vi "Connector Pane.vi"(8 "error in (no error)":errorcluster, 10 "Wire Middle? (F)":bool, 11 "VI Refnum in":refnum<vi>) -> (0 "error out":errorcluster, 3 "VI Refnum out":refnum<vi>)   [LabVIEW 2019, in "Builtins.lvlib"]
doc: "Wires the selected front panel controls and indicators to the connector pane ordered top-to-bottom then left-to-right respectively. Error In and Error Out terminals are wired to the bottom-left and bottom-right. All control terminals are set to Required inputs.\n\nCreated by: Ryan Pacini"
uses:
  Builtins.lvlib
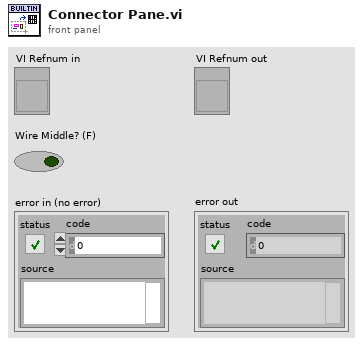
[diagram p1: front panel]
types:
  T1 = cluster{"Top":i16, "Left":i16, "Control":refnum<vi>}
  T2 = enum16{"Invalid Wire Rule", "Required", "Recommended", "Optional", "Dynamic Dispatch"}
  T3 = typedef "LVRectTypeDef.ctl" = cluster{"Left":i16, "Top":i16, "Right":i16, "Bottom":i16}
  T4 = cluster{"Top":i16, "Left":i16, "Control":refnum<vi>}[]
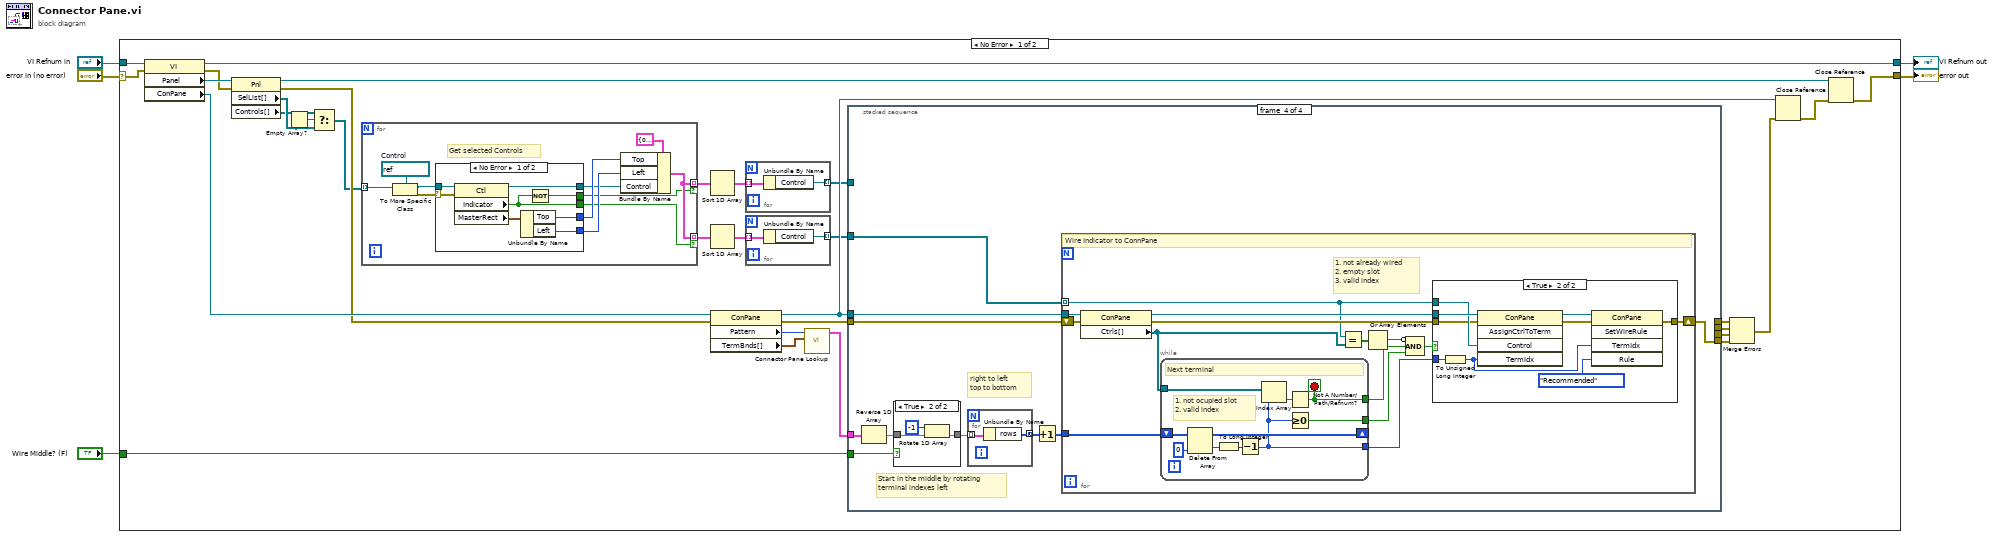
[diagram p0: block diagram]
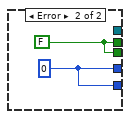
[diagram p2: hidden frame]
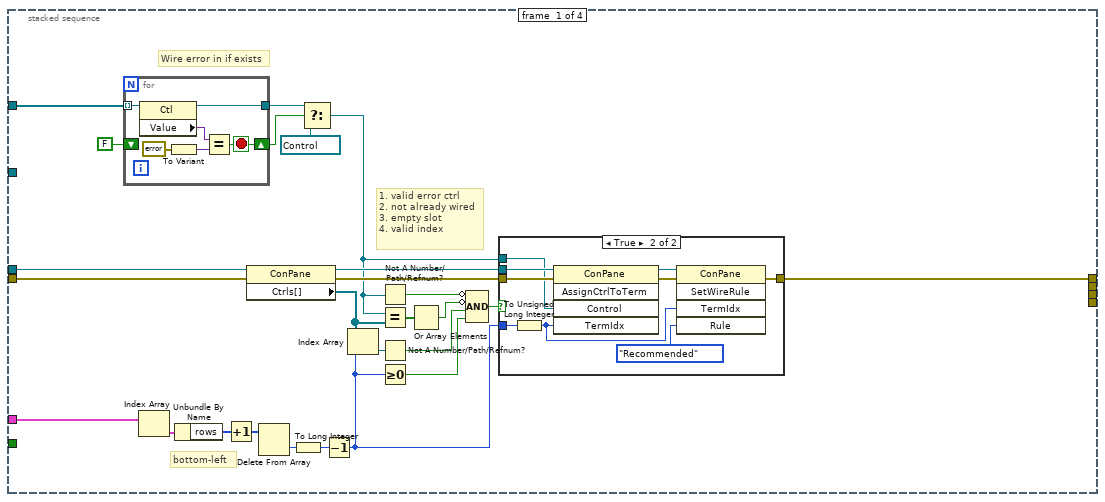
[diagram p3: hidden frame]
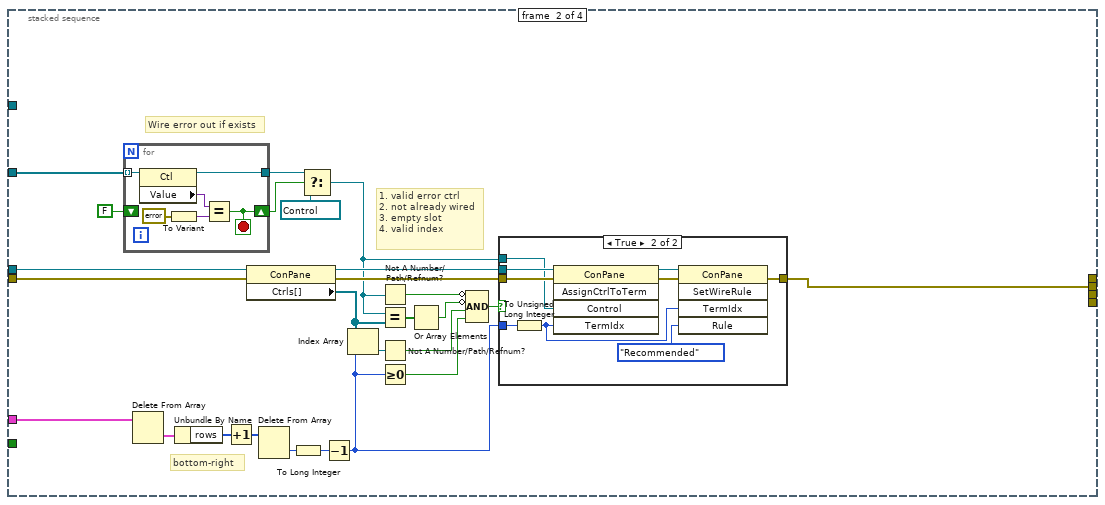
[diagram p5: hidden frame]
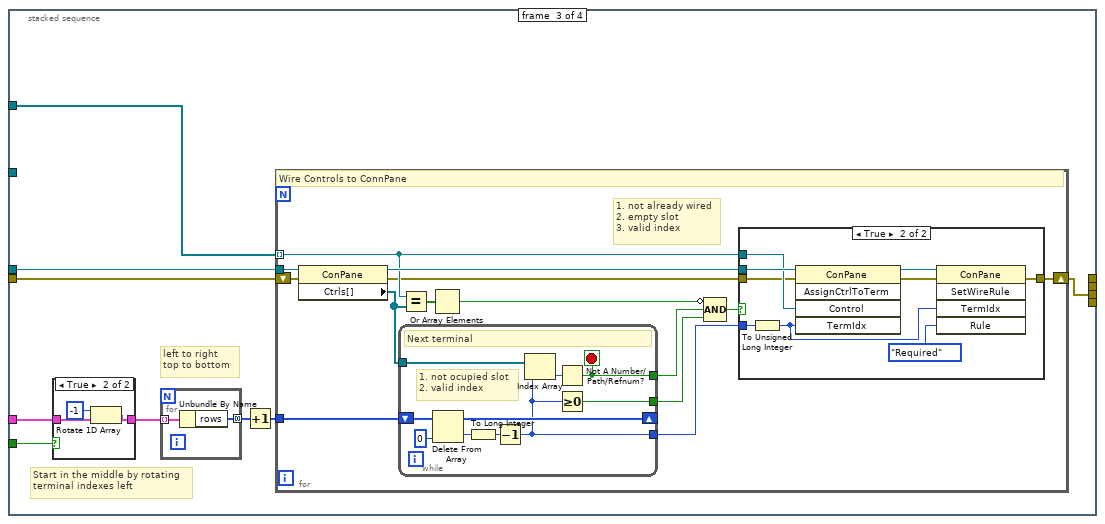
[diagram p7: hidden frame]
diagram:
  n1 = case shown="No Error" "error in (no error)" {
    selector: "error in (no error)" -> [w35 w245]
    tunnel: [w32 w246] -> w5
    tunnel: "VI Refnum in" -> [w36 w246]
    tunnel: [w18 w245] -> w2
    tunnel: "Wire Middle? (F)" -> [w6 _]
    frame No Error {
      n2 = property on="Property Node" class="VI"(reference=w36, error in=w35) -> (reference out=w32:refnum<vi>, error out=w33:errorcluster, "Panel"=w34:refnum<vi>, "ConPane"=w27:refnum<vi>)
      n3 = property on="Property Node" class="Pnl"(reference=w34, error in=w33) -> (reference out=w20:refnum<vi>, error out=w25:errorcluster, "SelList[]"=w10:refnum<vi>[], "Controls[]"=w9:refnum<vi>[])
      n4 = Empty Array?(array=w10) -> (empty?=w11:bool)
      n5 = Select(t=w9, s=w11, f=w10) -> (s? t:f=w8:refnum<vi>[])
      n6 = for {
        tunnel: w8 -> [w51] mode=indexing
        tunnel: [w46] -> w31 mode=indexing if=w43
        tunnel: [w46] -> w30 mode=indexing if=w42
        w50 = refnum<vi> refnum  # Control
        # "Get selected Controls"
        n7 = To More Specific Class(target class=w50, reference=w51) -> (specific class reference=w48:refnum<vi>, error out=w49:errorcluster)  [unwired: 1 in]
        n8 = case shown="No Error" w49 {
          selector: w49 -> [w52 _]
          tunnel: w48 -> [w59 _]
          tunnel: [w55 w61] -> w42
          tunnel: [w57 _] -> w41
          tunnel: [w56 w60] -> w47
          tunnel: [w54 w61] -> w43
          tunnel: [w53 w60] -> w44
          frame No Error {
            n9 = property class="Ctl"(reference=w59, error in=w52) -> (reference out=w57:refnum<vi>, "Indicator"=w55:bool, "MasterRect"=w58:T3)  [unwired: 1 out]
            n10 = Unbundle By Name(w58) -> ("Top"=w56:i16, "Left"=w53:i16)
            n11 = Not(x=w55) -> (.not. x?=w54:bool)
          }
          frame Error {
            w60 = i16 0 ("Top")
            w61 = FALSE
          }
        }
        n12 = Bundle By Name(cluster=T1 {"Top"=0, "Left"=0, "Control"=refnum}, "Top"=w47, "Left"=w44, "Control"=w41) -> (w46:T1)
      }
      n13 = Sort 1D Array(array=w31) -> (sorted array=w17:T4)
      n14 = Sort 1D Array(array=w30) -> (sorted array=w15:T4)
      n15 = property class="ConPane"(reference=w27, error in=w25) -> (reference out=w21:refnum<vi>, error out=w26:errorcluster, "Pattern"=w29:u32, "TermBnds[]"=w28:T3[])
      n16 = for {
        tunnel: w17 -> [w40] mode=indexing
        tunnel: [w39] -> w16 mode=indexing
        n17 = Unbundle By Name(w40) -> ("Control"=w39:refnum<vi>)
      }
      n18 = for {
        tunnel: w15 -> [w38] mode=indexing
        tunnel: [w37] -> w14 mode=indexing
        n19 = Unbundle By Name(w38) -> ("Control"=w37:refnum<vi>)
      }
      n20 = call "Connector Pane Lookup.vi"("TermBnds"=w28, "Pattern"=w29) -> ("columns"=w7:cluster{"rows":u8[]}[])  [unwired: 9 in]
      n21 = stacked-sequence {
        tunnel: w16 -> [w84 _ w150 _]
        tunnel: w7 -> [w66 w107 w148 w198]
        tunnel: w21 -> [w73 w117 w154 w204]
        tunnel: w14 -> [_ w105 _ w200]
        tunnel: w26 -> [w75 w118 w152 w202]
        tunnel: [_ _ w151 _] -> w24
        tunnel: [_ _ _ w199] -> w23
        tunnel: [_ w104 _ _] -> w13
        tunnel: [w62 _ _ _] -> w12
        tunnel: w6 -> [_ _ w147 w195]
        frame #0 {
          # "bottom-left"
          # "1. valid error ctrl\n2. not already wired\n3. empty slot\n4. valid index"
          # "Wire error in if exists"
          n22 = for {
            tunnel: w84 -> [w103] mode=indexing
            tunnel: [w99] -> w86
            shift-right: [w98] -> w87
            shift-left: FALSE -> [_]
            stop <- w98 stop-if-true
            n23 = property class="Ctl"(reference=w103) -> (reference out=w99:refnum<vi>, "Value"=w102:variant)  [unwired: 1 in, 1 out]
            n24 = To Variant(anything=errorcluster {"status"=FALSE, "code"=0, "source"=""} ("error in (no error)")) -> (Variant=w100:variant)
            n25 = Equal?(x=w102, y=w100) -> (x = y?=w98:bool)
          }
          n26 = Index Array(array=w66) -> (element=w74:cluster{"rows":u8[]})  [unwired: 1 in]
          n27 = Unbundle By Name(w74) -> ("rows"=w68:u8[])
          n28 = Increment(x=w68) -> (x+1=w65:u8[])
          n29 = property class="ConPane"(reference=w73, error in=w75) -> (reference out=w72:refnum<vi>, error out=w71:errorcluster, "Ctrls[]"=w79:refnum<vi>[])
          n30 = Delete From Array(array=w65) -> (deleted portion=w81:u8)  [unwired: 2 in, 1 out]
          n31 = To Long Integer(number=w81) -> (32bit integer=w67:i32)
          n32 = Select(t=w86, s=w87, f=refnum<vi> refnum) -> (s? t:f=w64:refnum<vi>)
          n33 = Decrement(x=w67) -> (x-1=w70:i32)
          n34 = Index Array(array=w79, index=w70) -> (element=w82:refnum<vi>)
          n35 = Not A Number/Path/Refnum?(number/path/refnum=w64) -> (NaN/Path/Refnum?=w63:bool)
          n36 = Equal?(x=w64, y=w79) -> (x = y?=w78:bool[])
          n37 = Not A Number/Path/Refnum?(number/path/refnum=w82) -> (NaN/Path/Refnum?=w80:bool)
          n38 = Greater Or Equal To 0?(x=w70) -> (x >= 0?=w76:bool)
          n39 = Or Array Elements(Boolean array=w78) -> (logical OR=w77:bool)
          n40 = Compound Arithmetic op=AND(invert w63, invert w77, w80, w76) -> (w69:bool)
          n41 = case shown="True" w69 {
            tunnel: w72 -> [_ w97]
            tunnel: w71 -> [w88 w96]
            tunnel: w70 -> [_ w95]
            tunnel: w64 -> [_ w94]
            tunnel: [w88 w91] -> w62
            frame False {
            }
            frame True {
              n42 = To Unsigned Long Integer(number=w95) -> (unsigned 32bit integer=w90:u32)
              n43 = invoke class="ConPane" method="AssignCtrlToTerm"(reference=w97, error in=w96, "Control"=w94, "TermIdx"=w90) -> (reference out=w93:refnum<vi>, error out=w92:errorcluster)  [unwired: 1 in, 3 out]
              n44 = invoke class="ConPane" method="SetWireRule"(reference=w93, error in=w92, "TermIdx"=w90, "Rule"=T2."Recommended") -> (error out=w91:errorcluster)  [unwired: 1 in, 4 out]
            }
          }
        }
        frame #1 {
          # "bottom-right"
          # "1. valid error ctrl\n2. not already wired\n3. empty slot\n4. valid index"
          # "Wire error out if exists"
          n45 = for {
            tunnel: w105 -> [w145] mode=indexing
            tunnel: [w141] -> w128
            shift-right: [w140] -> w129
            shift-left: FALSE -> [_]
            stop <- w140 stop-if-true
            n46 = property class="Ctl"(reference=w145) -> (reference out=w141:refnum<vi>, "Value"=w144:variant)  [unwired: 1 in, 1 out]
            n47 = To Variant(anything=errorcluster {"status"=FALSE, "code"=0, "source"=""} ("error in (no error)")) -> (Variant=w142:variant)
            n48 = Equal?(x=w144, y=w142) -> (x = y?=w140:bool)
          }
          n49 = Delete From Array(array=w107) -> (deleted portion=w106:cluster{"rows":u8[]})  [unwired: 2 in, 1 out]
          n50 = Unbundle By Name(w106) -> ("rows"=w112:u8[])
          n51 = Increment(x=w112) -> (x+1=w110:u8[])
          n52 = property class="ConPane"(reference=w117, error in=w118) -> (reference out=w116:refnum<vi>, error out=w115:errorcluster, "Ctrls[]"=w122:refnum<vi>[])
          n53 = Delete From Array(array=w110) -> (deleted portion=w124:u8)  [unwired: 2 in, 1 out]
          n54 = To Long Integer(number=w124) -> (32bit integer=w111:i32)
          n55 = Select(t=w128, s=w129, f=refnum<vi> refnum) -> (s? t:f=w109:refnum<vi>)
          n56 = Decrement(x=w111) -> (x-1=w114:i32)
          n57 = Index Array(array=w122, index=w114) -> (element=w125:refnum<vi>)
          n58 = Not A Number/Path/Refnum?(number/path/refnum=w109) -> (NaN/Path/Refnum?=w108:bool)
          n59 = Equal?(x=w109, y=w122) -> (x = y?=w121:bool[])
          n60 = Not A Number/Path/Refnum?(number/path/refnum=w125) -> (NaN/Path/Refnum?=w123:bool)
          n61 = Greater Or Equal To 0?(x=w114) -> (x >= 0?=w119:bool)
          n62 = Or Array Elements(Boolean array=w121) -> (logical OR=w120:bool)
          n63 = Compound Arithmetic op=AND(invert w108, invert w120, w123, w119) -> (w113:bool)
          n64 = case shown="True" w113 {
            tunnel: w116 -> [_ w139]
            tunnel: w115 -> [w130 w138]
            tunnel: w114 -> [_ w137]
            tunnel: w109 -> [_ w136]
            tunnel: [w130 w134] -> w104
            frame False {
            }
            frame True {
              n65 = To Unsigned Long Integer(number=w137) -> (unsigned 32bit integer=w131:u32)
              n66 = invoke class="ConPane" method="AssignCtrlToTerm"(reference=w139, error in=w138, "Control"=w136, "TermIdx"=w131) -> (reference out=w133:refnum<vi>, error out=w135:errorcluster)  [unwired: 1 in, 3 out]
              n67 = invoke class="ConPane" method="SetWireRule"(reference=w133, error in=w135, "TermIdx"=w131, "Rule"=T2."Recommended") -> (error out=w134:errorcluster)  [unwired: 1 in, 4 out]
            }
          }
        }
        frame #2 {
          # "Start in the middle by rotating\nterminal indexes left"
          # "left to right\ntop to bottom"
          n68 = case shown="True" w147 {
            tunnel: [w155 w158] -> w146
            tunnel: w148 -> [w155 w157]
            frame False {
            }
            frame True {
              n69 = Rotate 1D Array(1:w157, 2:-1 ("n")) -> (0:w158:cluster{"rows":u8[]}[])
            }
          }
          n70 = for {
            tunnel: w146 -> [w194] mode=indexing
            tunnel: [w193] -> w149 mode=concatenating
            n71 = Unbundle By Name(w194) -> ("rows"=w193:u8[])
          }
          n72 = Increment(x=w149) -> (x+1=w153:u8[])
          n73 = for {
            tunnel: w150 -> [w168] mode=indexing
            shift-right: [w164] -> w151
            shift-left: w152 -> [w163]
            tunnel: w154 -> [w172]
            tunnel: w153 -> [w171]
            # "1. not already wired\n2. empty slot\n3. valid index"
            # "Wire Controls to ConnPane"
            n74 = property class="ConPane"(reference=w172, error in=w163) -> (reference out=w170:refnum<vi>, error out=w165:errorcluster, "Ctrls[]"=w159:refnum<vi>[])
            n75 = while {
              tunnel: [w177] -> w162
              tunnel: [w173] -> w161
              tunnel: [w175] -> w160
              tunnel: w159 -> [w174]
              shift-right: [w180] -> _
              shift-left: w171 -> [w182]
              stop <- w173 stop-if-true
              # "1. not ocupied slot\n2. valid index"
              # "Next terminal"
              n76 = Delete From Array(array=w182, index=0) -> (deleted portion=w178:u8, array with subset deleted=w180:u8[])  [unwired: 1 in]
              n77 = To Long Integer(number=w178) -> (32bit integer=w176:i32)
              n78 = Decrement(x=w176) -> (x-1=w177:i32)
              n79 = Index Array(array=w174, index=w177) -> (element=w179:refnum<vi>)
              n80 = Not A Number/Path/Refnum?(number/path/refnum=w179) -> (NaN/Path/Refnum?=w173:bool)
              n81 = Greater Or Equal To 0?(x=w177) -> (x >= 0?=w175:bool)
            }
            n82 = Equal?(x=w168, y=w159) -> (x = y?=w167:bool[])
            n83 = Or Array Elements(Boolean array=w167) -> (logical OR=w166:bool)
            n84 = Compound Arithmetic op=AND(invert w166, w161, w160) -> (w169:bool)
            n85 = case shown="True" w169 {
              tunnel: w170 -> [_ w192]
              tunnel: w168 -> [_ w191]
              tunnel: w162 -> [_ w190]
              tunnel: w165 -> [w183 w189]
              tunnel: [w183 w186] -> w164
              frame False {
              }
              frame True {
                n86 = To Unsigned Long Integer(number=w190) -> (unsigned 32bit integer=w184:u32)
                n87 = invoke class="ConPane" method="AssignCtrlToTerm"(reference=w192, error in=w189, "Control"=w191, "TermIdx"=w184) -> (reference out=w185:refnum<vi>, error out=w187:errorcluster)  [unwired: 1 in, 3 out]
                n88 = invoke class="ConPane" method="SetWireRule"(reference=w185, error in=w187, "TermIdx"=w184, "Rule"=T2."Required") -> (error out=w186:errorcluster)  [unwired: 1 in, 4 out]
              }
            }
          }
        }
        frame #3 {
          # "Start in the middle by rotating\nterminal indexes left"
          # "right to left\ntop to bottom"
          n89 = Reverse 1D Array(array=w198) -> (reversed array=w197:cluster{"rows":u8[]}[])
          n90 = case shown="True" w195 {
            tunnel: [w205 w208] -> w196
            tunnel: w197 -> [w205 w207]
            frame False {
            }
            frame True {
              n91 = Rotate 1D Array(1:w207, 2:-1 ("n")) -> (0:w208:cluster{"rows":u8[]}[])
            }
          }
          n92 = for {
            tunnel: w196 -> [w244] mode=indexing
            tunnel: [w243] -> w201 mode=concatenating
            n93 = Unbundle By Name(w244) -> ("rows"=w243:u8[])
          }
          n94 = Increment(x=w201) -> (x+1=w203:u8[])
          n95 = for {
            tunnel: w200 -> [w212] mode=indexing
            shift-right: [w209] -> w199
            shift-left: w202 -> [w218]
            tunnel: w204 -> [w222]
            tunnel: w203 -> [w221]
            # "1. not already wired\n2. empty slot\n3. valid index"
            # "Wire Indicator to ConnPane"
            n96 = property class="ConPane"(reference=w222, error in=w218) -> (reference out=w213:refnum<vi>, error out=w214:errorcluster, "Ctrls[]"=w215:refnum<vi>[])
            n97 = while {
              tunnel: [w237] -> w210
              tunnel: [w233] -> w217
              tunnel: [w235] -> w216
              tunnel: w215 -> [w234]
              shift-right: [w240] -> _
              shift-left: w221 -> [w242]
              stop <- w233 stop-if-true
              # "1. not ocupied slot\n2. valid index"
              # "Next terminal"
              n98 = Delete From Array(array=w242, index=0) -> (deleted portion=w238:u8, array with subset deleted=w240:u8[])  [unwired: 1 in]
              n99 = To Long Integer(number=w238) -> (32bit integer=w236:i32)
              n100 = Decrement(x=w236) -> (x-1=w237:i32)
              n101 = Index Array(array=w234, index=w237) -> (element=w239:refnum<vi>)
              n102 = Not A Number/Path/Refnum?(number/path/refnum=w239) -> (NaN/Path/Refnum?=w233:bool)
              n103 = Greater Or Equal To 0?(x=w237) -> (x >= 0?=w235:bool)
            }
            n104 = Equal?(x=w212, y=w215) -> (x = y?=w220:bool[])
            n105 = Or Array Elements(Boolean array=w220) -> (logical OR=w219:bool)
            n106 = Compound Arithmetic op=AND(invert w219, w217, w216) -> (w211:bool)
            n107 = case shown="True" w211 {
              tunnel: w213 -> [_ w232]
              tunnel: w212 -> [_ w231]
              tunnel: w210 -> [_ w230]
              tunnel: w214 -> [w223 w229]
              tunnel: [w223 w226] -> w209
              frame False {
              }
              frame True {
                n108 = To Unsigned Long Integer(number=w230) -> (unsigned 32bit integer=w224:u32)
                n109 = invoke class="ConPane" method="AssignCtrlToTerm"(reference=w232, error in=w229, "Control"=w231, "TermIdx"=w224) -> (reference out=w225:refnum<vi>, error out=w227:errorcluster)  [unwired: 1 in, 3 out]
                n110 = invoke class="ConPane" method="SetWireRule"(reference=w225, error in=w227, "TermIdx"=w224, "Rule"=T2."Recommended") -> (error out=w226:errorcluster)  [unwired: 1 in, 4 out]
              }
            }
          }
        }
      }
      n111 = Merge Errors(w12, w13, w24, w23) -> (w22:errorcluster)
      n112 = Close Reference(reference=w21, error in (no error)=w22) -> (error out=w19:errorcluster)
      n113 = Close Reference(reference=w20, error in (no error)=w19) -> (error out=w18:errorcluster)
    }
    frame Error {
    }
  }
  "VI Refnum out" <- w5
  "error out" <- w2
